vi "Diff_Drive_System_Acquire.vi"(6 "FPGA_Time_Seconds":dbl, 11 "DiffDriveDeviceRefs":T1 {"GyroDevRef"."Sample Rate" min=0.25 max=100.0 step=0.25}) -> (2 "Right Speed":dbl, 3 "Left Speed":dbl)   [LabVIEW 2019]
uses:
  Diff_Drive_System_Globals.vi
  <vilib>/Rock Robotics/SystemInterfaces/AI/FPGA_AIGyroChannel.ctl
  <vilib>/Rock Robotics/WPI/ThirdParty/JAS_Junk/TrajLib/Trajectory_Library.lvlib
  <vilib>/Rock Robotics/SystemInterfaces/spilib/spi_bus.ctl
  <vilib>/Rock Robotics/SystemInterfaces/AI/FPGA_AIChannel.ctl
  <vilib>/Rock Robotics/WPI/Gyro/WPI_GyroDevRef.ctl
  <vilib>/Rock Robotics/SystemInterfaces/Encoder/FPGA_EncoderIdx.ctl
  <vilib>/Rock Robotics/WPI/Encoder/WPI_EncoderType.ctl
  <vilib>/Rock Robotics/SystemInterfaces/Counter/FPGA_CounterCtrSystemIndex.ctl
  <vilib>/Rock Robotics/WPI/Encoder/WPI_EncoderDevRef.ctl
  <vilib>/Rock Robotics/SystemInterfaces/DIO/FPGA_DIOPWMChannel.ctl
  <vilib>/Rock Robotics/WPI/PWM/WPI_PWMDeadband.ctl
  <vilib>/Rock Robotics/WPI/MotorControl/WPI_MotorControlType.ctl
  <vilib>/Rock Robotics/SystemInterfaces/DIO/FPGA_DIOChannel.ctl
  <vilib>/Rock Robotics/WPI/MotorControl/WPI_MotorControlDeviceRef.ctl
  <vilib>/Rock Robotics/WPI/RobotDrive/WPI_RobotDriveDevRef.ctl
  Diff_Drive_System_Device_Refs.ctl
panel:
  # "Analog"
  # "XRS"
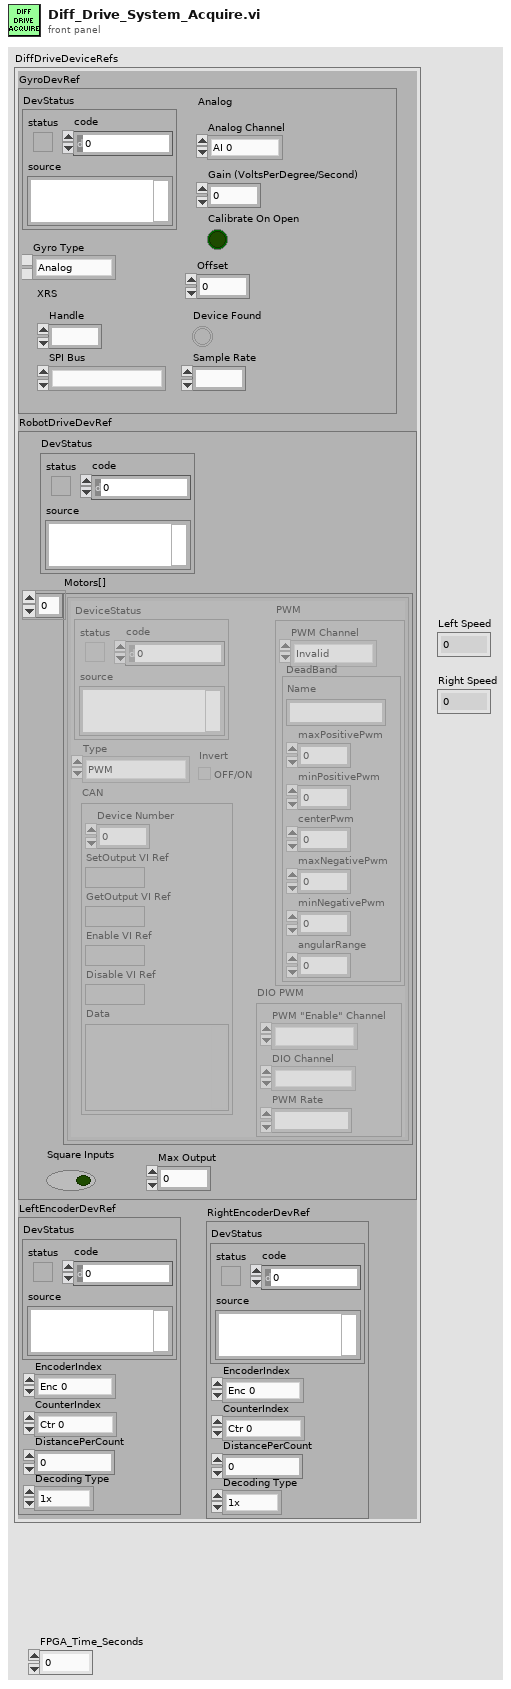
[diagram p1: front panel]
types:
  T1 = typedef "Diff_Drive_System_Device_Refs.ctl" = cluster{"GyroDevRef":T2, "RobotDriveDevRef":T5, "LeftEncoderDevRef":T11, "RightEncoderDevRef":T11}
  T2 = typedef "WPI_GyroDevRef.ctl" = cluster{"DevStatus":errorcluster, "Analog Channel":T3, "Gain (VoltsPerDegree/Second)":dbl, "Gyro Type":enum16{"Analog", "XRS450"}, "Handle":i32, "SPI Bus":T4, "Device Found":bool, "Sample Rate":dbl, "Calibrate On Open":bool, "Offset":dbl}
  T3 = typedef "FPGA_AIChannel.ctl" = enum8{"AI 0", "AI 1", "AI 2", "AI 3", "AI MXP 0", "AI MXP 1", "AI MXP 2", "AI MXP 3", "Invalid"}
  T4 = typedef "spi_bus.ctl" = enum16{"SPI On-Board, CS0", "SPI On-Board, CS1", "SPI On-Board, CS2", "SPI On-Board, CS3", "SPI MXP", "Invalid"}
  T5 = typedef "WPI_RobotDriveDevRef.ctl" = cluster{"DevStatus":errorcluster, "Motors[]":T6[], "Square Inputs":bool, "Max Output":dbl}
  T6 = typedef "WPI_MotorControlDeviceRef.ctl" = cluster{"DeviceStatus":errorcluster, "Type":T7, "PWM":cluster{"PWM Channel":T8, "DeadBand":T9}, "CAN":cluster{"Device Number":u8, "SetOutput VI Ref":variant, "GetOutput VI Ref":variant, "Enable VI Ref":variant, "Disable VI Ref":variant, "Data":variant}, "Invert":bool, "DIO PWM":cluster{"PWM \"Enable\" Channel":T8, "DIOChannel":T10, "PWM Rate":dbl}}
  T7 = typedef "WPI_MotorControlType.ctl" = enum16{"PWM", "CAN", "DIO PWM"}
  T8 = typedef "FPGA_DIOPWMChannel.ctl" = enum8{"PWM 0", "PWM 1", "PWM 2", "PWM 3", "PWM 4", "PWM 5", "PWM 6", "PWM 7", "PWM 8", "PWM 9", "PWM MXP 0", "PWM MXP 1", "PWM MXP 2", "PWM MXP 3", "PWM MXP 4", "PWM MXP 5", "PWM MXP 6", "PWM MXP 7", "PWM MXP 8", "PWM MXP 9", "Invalid"}
  T9 = typedef "WPI_PWMDeadband.ctl" = cluster{"Name":string, "maxPositivePwm":i32, "minPositivePwm":i32, "centerPwm":i32, "maxNegativePwm":i32, "minNegativePwm":i32, "angularRange":u16}
  T10 = typedef "FPGA_DIOChannel.ctl" = enum8{"DIO 0", "DIO 1", "DIO 2", "DIO 3", "DIO 4", "DIO 5", "DIO 6", "DIO 7", "DIO 8", "DIO 9", "DIO MXP 0", "DIO MXP 1", "DIO MXP 2", "DIO MXP 3", "DIO MXP 4", "DIO MXP 5", "DIO MXP 6", "DIO MXP 7", "DIO MXP 8", "DIO MXP 9", "DIO MXP 10", "DIO MXP 11", "DIO MXP 12", "DIO MXP 13", "DIO MXP 14", "DIO MXP 15", "SPI Port CS1", "SPI Port CS2", "SPI Port CS3", "SPI Port MISO", "SPI Port MOSI", "Invalid"}
  T11 = typedef "WPI_EncoderDevRef.ctl" = cluster{"DevStatus":errorcluster, "EncoderIndex":T12, "CounterIndex":T13, "DistancePerCount":dbl, "Decoding Type":T14}
  T12 = typedef "FPGA_EncoderIdx.ctl" = enum8{"Enc 0", "Enc 1", "Enc 2", "Enc 3", "Enc 4", "Enc 5", "Enc 6", "Enc 7", "Invalid"}
  T13 = typedef "FPGA_CounterCtrSystemIndex.ctl" = enum8{"Ctr 0", "Ctr 1", "Ctr 2", "Ctr 3", "Ctr 4", "Ctr 5", "Ctr 6", "Ctr 7", "Invalid"}
  T14 = typedef "WPI_EncoderType.ctl" = enum16{"1x", "2x", "4x"}
  T15 = enum16{"Moving Average", "Low Pass 1st Order Butterworth", "Low Pass 2nd Order Butterworth", "High Pass 1st Order Butterworth", "High Pass 2nd Order Butterworth"}
  T16 = typedef "FPGA_AIGyroChannel.ctl" = enum8{"AI 0", "AI 1", "Invalid"}
  T17 = cluster{">angleX":dbl, ">angleY":dbl, ">angleZ":dbl}
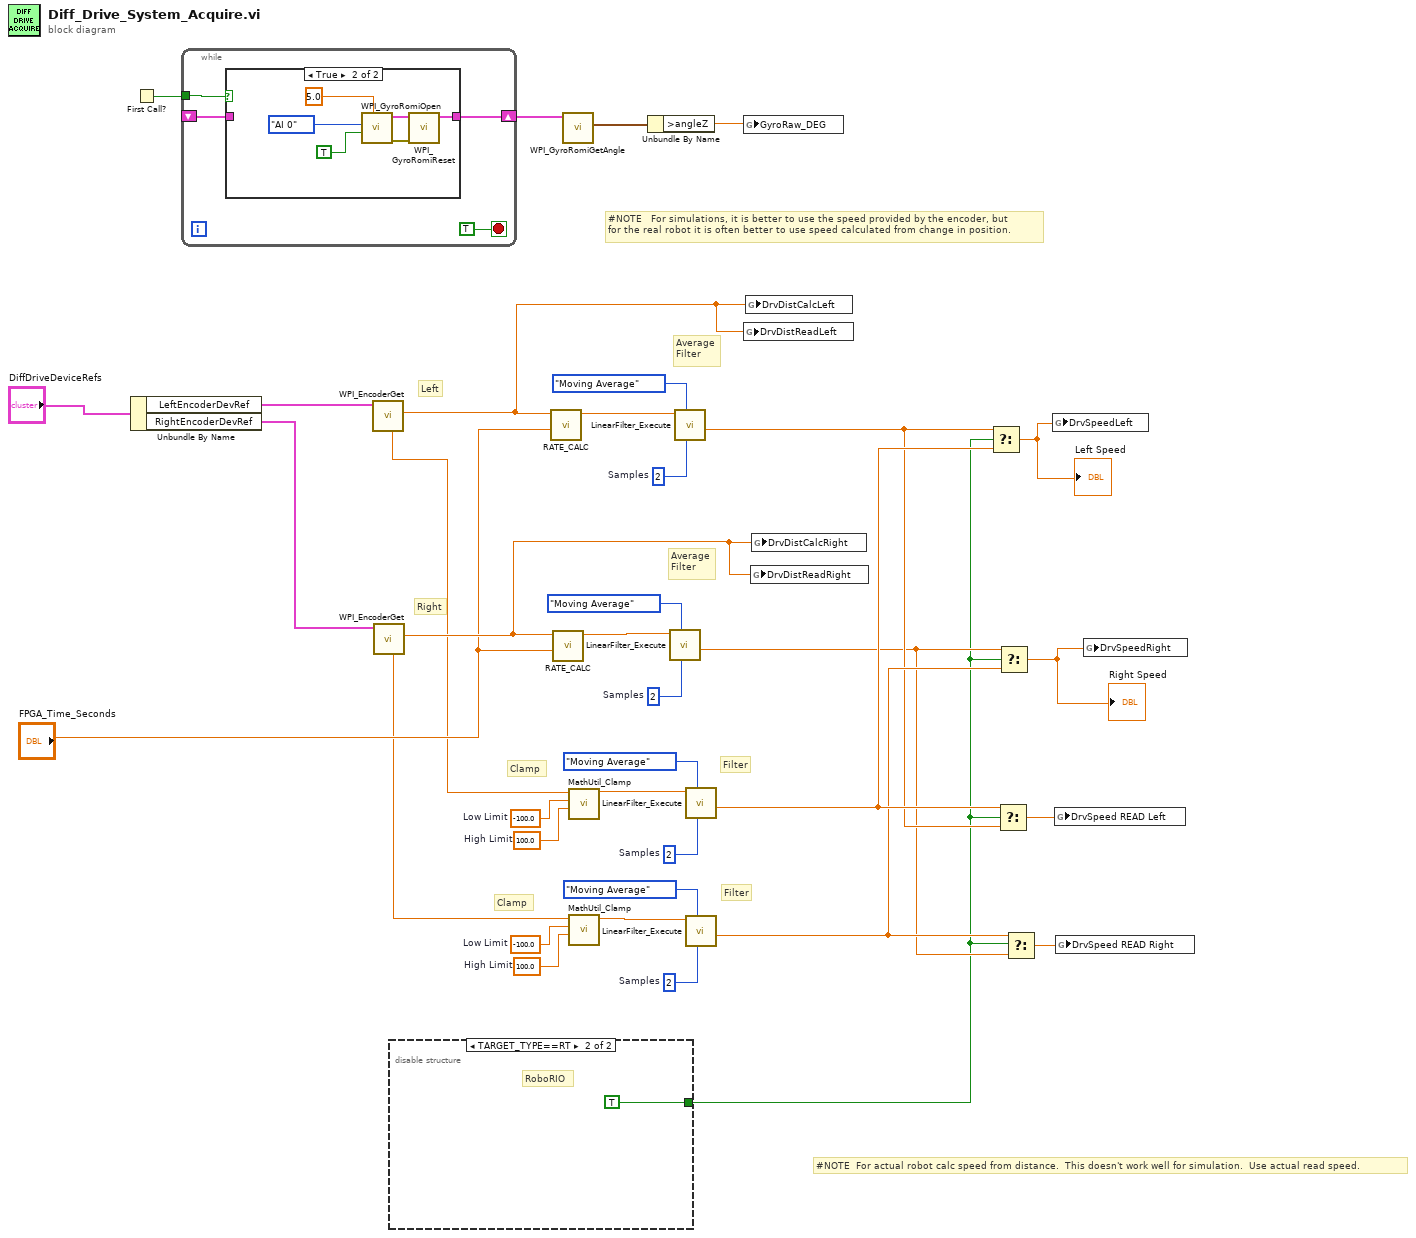
[diagram p0: block diagram]
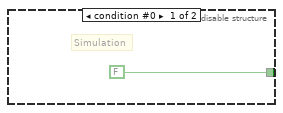
[diagram p2: hidden frame]
diagram:
  w6 = 100.0  # High Limit
  w5 = -100.0  # Low Limit
  w8 = 100.0  # High Limit
  w7 = -100.0  # Low Limit
  w19 = 2  # Samples
  w21 = 2  # Samples
  w24 = 2  # Samples
  w27 = 2  # Samples
  # "Filter"
  # "Filter"
  # "Clamp"
  # "Clamp"
  # "#NOTE  For actual robot calc speed from distance.  This doesn't work well for simulation.  Use actual read speed."
  # "#NOTE   For simulations, it is better to use the speed provided by the encoder, but\nfor the real robot it is often better to use speed calculated from change in position."
  # "Average\nFilter"
  # "Average\nFilter"
  # "Right"
  # "Left"
  n1 = Unbundle By Name("DiffDriveDeviceRefs") -> ("LeftEncoderDevRef"=w36:T11, "RightEncoderDevRef"=w35:T11)
  n2 = First Call?() -> (First Call?: T/F=w34:bool)
  n3 = while {
    tunnel: w34 -> [w41]
    shift-right: [w39] -> w33
    shift-left: _ -> [w38]
    stop <- TRUE stop-if-true
    n4 = case shown="True" w41 {
      tunnel: [w42 w43] -> w39
      tunnel: w38 -> [w42 _]
      frame False {
      }
      frame True {
        n5 = call <vilib>:"WPI_GyroRomiOpen.vi"("Calibration Time (s)"=5.0, "Calibrate On Open"=TRUE, "Analog Channel"=FPGA_AIGyroChannel."AI 0") -> ("error out"=w45:errorcluster, "GyroDevRef"=w44:T2)  [unwired: 7 in]
        n6 = call <vilib>:"WPI_GyroRomiReset.vi"("error in (no error)"=w45, "GyroDevRef"=w44) -> ("GyroDevRef"=w43:T2)  [unwired: 8 in, 1 out]
      }
    }
  }
  n7 = call <vilib>:"WPI_EncoderGet.vi"("EncoderDevRef"=w36) -> ("Distance"=w30:dbl, "Rate"=w2:dbl)  [unwired: 5 in, 4 out]
  n8 = call <vilib>:"WPI_EncoderGet.vi"("EncoderDevRef"=w35) -> ("Distance"=w29:dbl, "Rate"=w1:dbl)  [unwired: 5 in, 4 out]
  n9 = disable-structure shown="TARGET_TYPE==RT" {
    disable-tunnel: [FALSE TRUE] -> w9
    frame condition #0 {
      # "Simulation"
    }
    frame condition #1 (active) {
      # "RoboRIO"
    }
  }
  n10 = call "RATE_CALC.vi"("Time"="FPGA_Time_Seconds", "Input"=w30) -> ("Output"=w25:dbl)  [unwired: 9 in]
  n11 = call "RATE_CALC.vi"("Time"="FPGA_Time_Seconds", "Input"=w29) -> ("Output"=w22:dbl)  [unwired: 9 in]
  n12 = call <vilib>:"WPI_GyroRomiGetAngle.vi"("GyroDevRef"=w33) -> ("Angle"=w32:T17)  [unwired: 6 in, 4 out]
  n13 = call <vilib>:"MathUtil_Clamp.vi"("High Limit"=w8, "Low Limit"=w7, "Value"=w2) -> ("Result"=w3:dbl)  [unwired: 8 in]
  n14 = call <vilib>:"MathUtil_Clamp.vi"("High Limit"=w6, "Low Limit"=w5, "Value"=w1) -> ("Result"=w4:dbl)  [unwired: 8 in]
  n15 = Unbundle By Name(w32) -> (">angleZ"=w31:dbl)
  n16 = call <vilib>:"LinearFilter_Execute.vi"("Samples"=w24, "Filter Type"=T15."Moving Average", "Input"=w22) -> ("Output"=w10:dbl)  [unwired: 7 in, 1 out]
  n17 = call <vilib>:"LinearFilter_Execute.vi"("Samples"=w27, "Filter Type"=T15."Moving Average", "Input"=w25) -> ("Output"=w11:dbl)  [unwired: 7 in, 1 out]
  n18 = call <vilib>:"LinearFilter_Execute.vi"("Samples"=w21, "Filter Type"=T15."Moving Average", "Input"=w3) -> ("Output"=w16:dbl)  [unwired: 7 in, 1 out]
  n19 = call <vilib>:"LinearFilter_Execute.vi"("Samples"=w19, "Filter Type"=T15."Moving Average", "Input"=w4) -> ("Output"=w12:dbl)  [unwired: 7 in, 1 out]
  n20 = global write "Diff_Drive_System_Globals.vi" "GyroRaw_DEG"(w31) -> ()
  n21 = global write "Diff_Drive_System_Globals.vi" "DrvDistReadLeft"(w30) -> ()
  n22 = global write "Diff_Drive_System_Globals.vi" "DrvDistCalcLeft"(w30) -> ()
  n23 = global write "Diff_Drive_System_Globals.vi" "DrvDistReadRight"(w29) -> ()
  n24 = global write "Diff_Drive_System_Globals.vi" "DrvDistCalcRight"(w29) -> ()
  n25 = Select(t=w11, s=w9, f=w16) -> (s? t:f=w17:dbl)
  "Left Speed" <- w17
  n26 = Select(t=w16, s=w9, f=w11) -> (s? t:f=w14:dbl)
  n27 = Select(t=w10, s=w9, f=w12) -> (s? t:f=w15:dbl)
  "Right Speed" <- w15
  n28 = Select(t=w12, s=w9, f=w10) -> (s? t:f=w13:dbl)
  n29 = global write "Diff_Drive_System_Globals.vi" "DrvSpeedLeft"(w17) -> ()
  n30 = global write "Diff_Drive_System_Globals.vi" "DrvSpeed READ Left"(w14) -> ()
  n31 = global write "Diff_Drive_System_Globals.vi" "DrvSpeed READ Right"(w13) -> ()
  n32 = global write "Diff_Drive_System_Globals.vi" "DrvSpeedRight"(w15) -> ()
